vi "Image_Processing_InvertingImage.vi"() -> ()   [LabVIEW 2015]
uses:
  <vilib>/picture/picture.llb/imagedata.ctl
panel:
  in  "output image":path
  out "new picture 2":picture
  out "new picture":picture
  out "image data":T1
  in  "Input Image":path
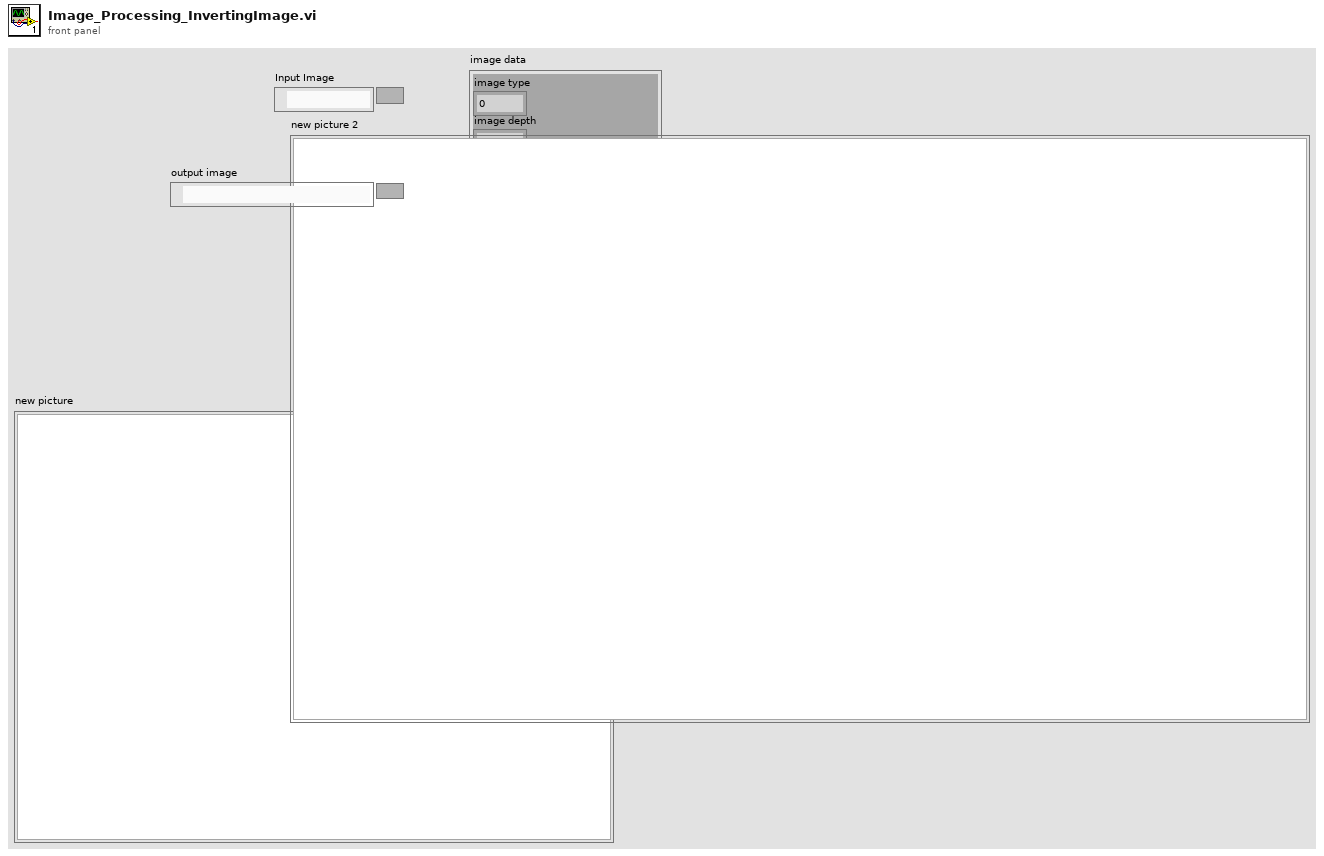
[diagram p1: front panel]
types:
  T1 = typedef "imagedata.ctl" = cluster{"image type":i32, "image depth":i32, "image":u8[], "mask":u8[], "colors":u32[], "Rectangle":cluster{"left":i16, "top":i16, "right":i16, "bottom":i16}}
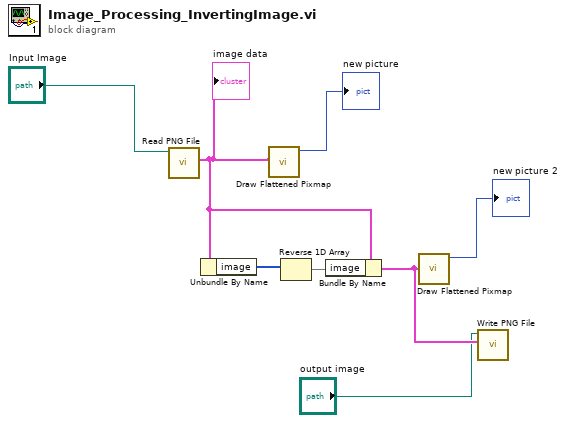
[diagram p0: block diagram]
diagram:
  n1 = call <vilib>:"Read PNG File.vi"("path to PNG file"="Input Image") -> ("image data"=w4:T1)  [unwired: 8 in, 2 out]
  "image data" <- w4
  n2 = Unbundle By Name(w4) -> ("image"=w6:u8[])
  n3 = call <vilib>:"Draw Flattened Pixmap.vi"("image data"=w4) -> ("new picture"=→"new picture":picture)  [unwired: 8 in]
  n4 = Reverse 1D Array(array=w6) -> (reversed array=w5:u8[])
  n5 = Bundle By Name(cluster=w4, "image"=w5) -> (w2:T1)
  n6 = call <vilib>:"Draw Flattened Pixmap.vi"("image data"=w2) -> ("new picture"=→"new picture 2":picture)  [unwired: 8 in]
  n7 = call <vilib>:"Write PNG File.vi"("image data"=w2, "path to PNG file"="output image") -> ()  [unwired: 8 in, 2 out]
